vi "getMotorNames.vi"(11 "DeviceName":string) -> (3 "elements":string[](array[string]))   [LabVIEW 2013]
uses:
  shared programs/MySQL/Preset Query Enum.ctl
  <userlib>/_OpenG.lib/array/array.llb/Filter 1D Array (String)__ogtk.vi
  <userlib>/_OpenG.lib/array/array.llb/Index 1D Array Elements (String)__ogtk.vi
  <userlib>/_OpenG.lib/array/array.llb/Remove Duplicates from 1D Array (String)__ogtk.vi
  <userlib>/_OpenG.lib/array/array.llb/Filter 1D Array with Scalar (String)__ogtk.vi
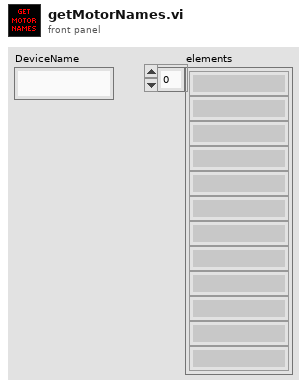
[diagram p1: front panel]
types:
  T1 = typedef "Preset Query Enum.ctl" = enum16{"Get Locations", "Get all IPs and MACs", "Get classes", "Get expt variables to set at scanstart for particular device", "Get expt devices and variables with start values", "Get expt devices and variables (with data to get)", "Get expt devices with data to get", "Get Expt devices and GUIs", "Get all devices basic properties", "Get Virtual Devices Core Info", "Get Expt names", "Get experiment basic properties", "Get experiment alarm variables", "Get MC Ports", "Get device network comm port", "Get devicetype lvclass path", "Get basic device properties", "Get Init Order", "Get all setable variables of a device", "Get device variable aliases", "Get force values of all settable variables", "Get all variables of a devicetype", "Get all variables of a device", "Get plotter details", "Get Saved Scans", "Get Scan Info", "GetGeneralGUIs", "Get expt for plotter", "Get plotter IDs from expt", "Get all devices", "Get all Virtual Devices", "Get variable and device info for Virtual Device", "GetItemLocatorIP", "Get IPs for GUIs", "Get DeviceType from Device", "GetLocalPortRange", "GetDevicePresetVariables", "Get Device Configuration", "GetAllPresetNames", "GetAllConfigurationNames", "GetPresetDeviceNames"}
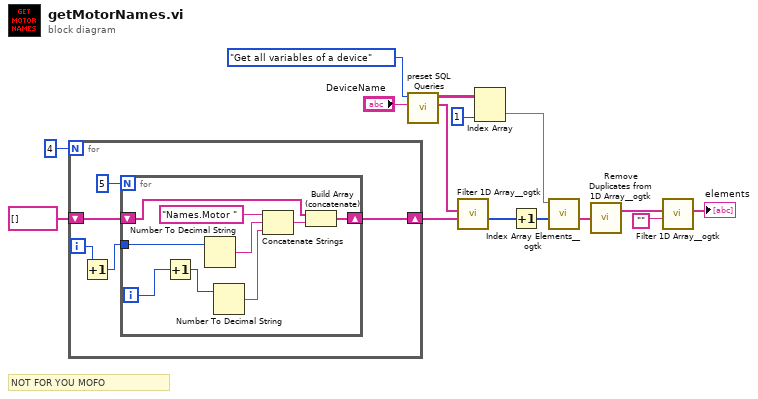
[diagram p0: block diagram]
diagram:
  # "NOT FOR YOU MOFO"
  n1 = for {
    N: 4 -> [_]
    shift-right: [w19] -> w10
    shift-left: string[] [] -> [w18]
    i -> [w17]
    n2 = Increment(x=w17) -> (x+1=w16:i32)
    n3 = for {
      N: 5 -> [_]
      tunnel: w16 -> [w29]
      shift-right: [w24] -> w19
      shift-left: w18 -> [w26]
      i -> [w22]
      n4 = Increment(x=w22) -> (x+1=w21:i32)
      n5 = Number To Decimal String(number=w29) -> (decimal integer string=w28:string)  [unwired: 1 in]
      n6 = Number To Decimal String(number=w21) -> (decimal integer string=w27:string)  [unwired: 1 in]
      n7 = Concatenate Strings("Names.Motor " ("string"), w28, w27) -> (w25:string)
      n8 = Build Array (concatenate)(w26, w25) -> (w24:string[])
    }
  }
  n9 = call "preset SQL Queries.vi"("Device/Devicetype name\n/Plotter.id/ScanName#"="DeviceName", "Preset Query"=Preset_Query_Enum."Get all variables of a device") -> ("1st column 1st data"=w7:string[], "data"=w11:string[][])  [unwired: 7 in, 1 out]
  n10 = call-poly <userlib>:"Filter 1D Array__ogtk.vi"("items to filter"=w10, "array"=w7) -> ("filtered item indices"=w14:i32[])  [unwired: 4 in, 1 out]
  n11 = Index Array(array=w11, index (col)=1 ("disabled index (col)")) -> (element=w13:string[])  [unwired: 1 in]
  n12 = Increment(x=w14) -> (x+1=w15:i32[])
  n13 = call-poly <userlib>:"Index Array Elements__ogtk.vi"("indices"=w15, "array"=w13) -> ("elements"=w1:string[])  [unwired: 9 in]
  n14 = call-poly <userlib>:"Remove Duplicates from 1D Array__ogtk.vi"("Input Array"=w1) -> ("Output Array"=w4:string[])  [unwired: 1 out]
  n15 = call-poly <userlib>:"Filter 1D Array__ogtk.vi"("items to filter"="", "array"=w4) -> ("filtered array"=→"elements":string[])  [unwired: 4 in, 1 out]
